vi "Configure Trigger (Communication - NRZ,MLT3).vi"(0 "VISA resource name":refnum<visa-resource-name>, 1 "Coding (0:NRZ)":u16(ring) items=["NRZ", "MLT3"], 2 "Standard (0:ATAG1)":u16(ring) items=["ATAG1"=0, "ATAG2"=1, "ATAG3"=2, "D1"=5, "D2"=6, "RATE32Mbit"=17, "RATE97Mbit"=18, "STS1"=25, "STS3"=26, "STM1E"=27, "FC133"=28, "FC266"=29, "FC531"=30, "FC1063"=31, "FC2125"=32, "FC4250"=33, "OC1"=34, "OC3"=35, "OC12"=36, "OC48"=37, "OC48_FEC"=38, "STM1E"=39, "ENET100"=40, "ENET1250"=41, "ENETXAUI"=42, "INF2_5G"=43, "FST"=44, "HST"=45, "FW1394BS400B"=46, "FW1394BS1600B"=47, "RIO_500M"=48, "RIO_750M"=49, "RIO_1G"=50, "RIO_1_5G"=51, "RIO_2G"=52, "RIO_SERIAL_1G"=53, "RIO_SERIAL_2G"=54, "RIO_SERIAL_3G"=55, "SAS1_5"=56, "SAS3_0"=57, "SFI5_2"=58, "STM0_HDBX"=59, "STM0_CMI"=60, "RATE32Mbit"=61, "RATE97Mbit"=62, "SFI5_3"=63, "VSROC192"=64, "TFI5_2"=65, "TFI5_3"=66, "PCIEXPRESS"=67, "VIDEO270"=68, "VIDEO360"=69, "VIDEO292M"=71, "Custom"=70], 3 "Bit Rate (1.544E6Mb/s)":dbl=1544000.0, 5 "Source (0:Channel1)":u16(ring) items=["Channel1", "Channel2", "Channel3", "Channel4"], 7 "Trigger Level (0V)":dbl, 9 "Source Type (0:Data)":u16(ring) items=["Data", "Clock", "Recovered"], 11 "error in (no error)":errorcluster, 12 "Clock Polarity (0:Positive)":u16(ring) items=["Positive", "Negative"]) -> (4 "VISA resource name out":refnum<visa-resource-name>, 15 "error out":errorcluster)   [LabVIEW 2012, in "Tektronix 7000 Series.lvlib"]
doc: "Configures Communication trigger settings for an oscilloscope.A trigger occurs when a communications signal is found. Supports MLT3 and NRZ encoded communications signals.\n\nTDS5000,TDS5000B series oscilloscopes don't support this trigger."
uses:
  Tektronix 7000 Series.lvlib
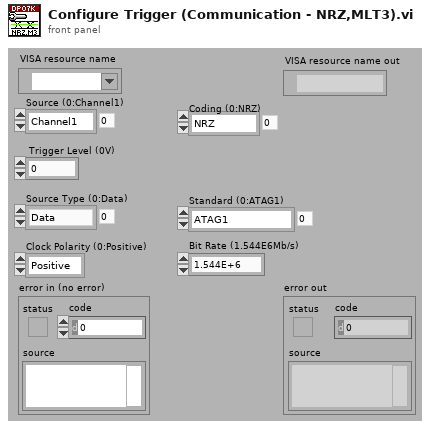
[diagram p1: front panel]
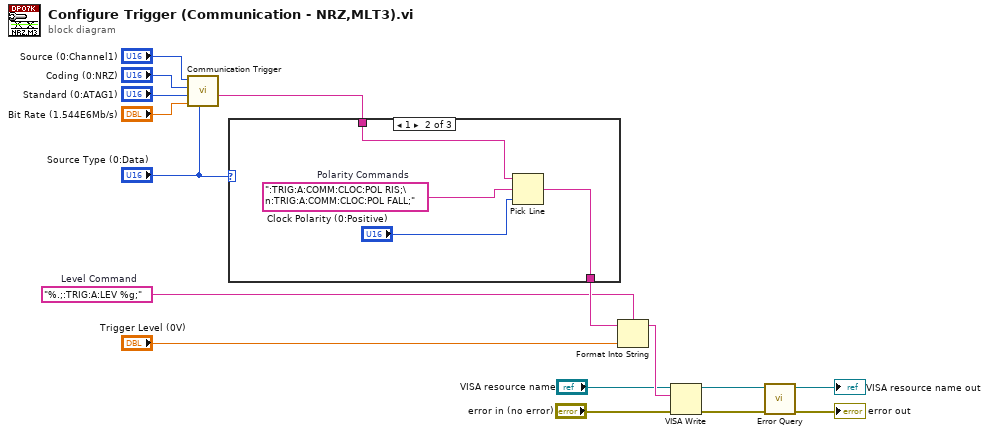
[diagram p0: block diagram]
diagram:
  w9 = "%.;:TRIG:A:LEV %g;"  # Level Command
  n1 = call "Communication Trigger.vi"("Source Type (0:Data)"="Source Type (0:Data)", "Bit Rate (1.544E6Mb/s)"="Bit Rate (1.544E6Mb/s)", "Standard (0:ATAG1)"="Standard (0:ATAG1)", "Coding (0:NRZ)"="Coding (0:NRZ)", "Source (0:Channel1)"="Source (0:Channel1)") -> ("Output String"=w11:string)  [unwired: 6 in]
  n2 = case shown="1" "Source Type (0:Data)" {
    tunnel: w11 -> [w17 w21 w22]
    tunnel: [w17 w18 w22] -> w10
    frame 0, Default {
    }
    frame 1 {
      w20 = ":TRIG:A:COMM:CLOC:POL RIS;\n:TRIG:A:COMM:CLOC:POL FALL;"  # Polarity Commands
      n3 = Pick Line(string ("")=w21, multi-line string=w20, line index="Clock Polarity (0:Positive)") -> (output string=w18:string)
    }
    frame 2 {
    }
  }
  n4 = Format Into String(format string=w9, initial string=w10, "Trigger Level (0V)") -> (resulting string=w5:string)  [unwired: 1 in, 1 out]
  n5 = VISA Write(VISA resource name="VISA resource name", write buffer=w5, error in (no error)="error in (no error)") -> (VISA resource name out=w6:refnum<visa-resource-name>, error out=w7:errorcluster)  [unwired: 1 out]
  n6 = call "Error Query.vi"("error in (no error)"=w7, "VISA resource name"=w6) -> ("error out"=→"error out":errorcluster, "VISA resource name out"=→"VISA resource name out":refnum<visa-resource-name>)  [unwired: 6 in, 2 out]
